vi "subVITest.vi"(11 "Particle Measurements (Pixels) (Particle Analysis 1)":dbl[][](array[numeric])) -> (3 "GREEN?":bool)   [LabVIEW 2017]
doc: "yeeeeeeeeeeeeeeeeeeeeeeee"
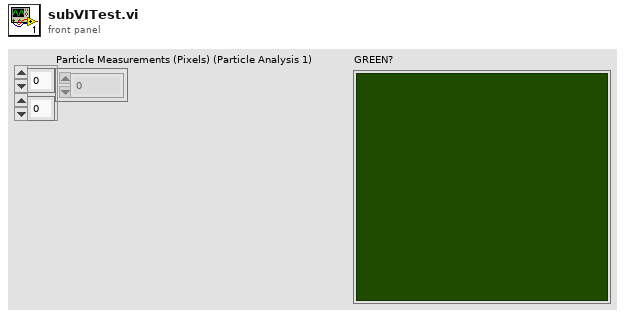
[diagram p1: front panel]
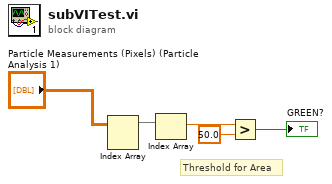
[diagram p0: block diagram]
diagram:
  # "Threshold for Area"
  n1 = Index Array(array="Particle Measurements (Pixels) (Particle Analysis 1)") -> (element=w1:dbl[])  [unwired: 2 in]
  n2 = Index Array(array=w1) -> (element=w2:dbl)  [unwired: 1 in]
  n3 = Greater?(x=w2, y=50.0) -> (0:→"GREEN?":bool)
